vi "CategoricalNB.vi"(8 "error in":errorcluster) -> (0 "error out":errorcluster, 3 "out":refnum<class "CategoricalNB.lvclass">)   [LabVIEW 2020]
doc: "Naive Bayes classifier for categorical features\n\n The categorical Naive Bayes classifier is suitable for classification with\n discrete features that are categorically distributed. The categories of\n each feature are drawn from a categorical distribution.\n\n Read more in the :ref:`User Guide <categorical_naive_bayes>`.\n\n Parameters\n ----------\n alpha : float, default=1.0\n Additive (Laplace/Lidstone) smoothing parameter\n (0 for no smoothing).\n\n fit_prior : bool, default=True\n Whether to learn class prior probabilities or not.\n If false, a uniform prior will be used.\n\n class_prior : array-like of shape (n_classes,), default=None\n Prior probabilities of the classes. If specified the priors are not\n adjusted according to the data.\n\n min_categories : int or array-like of shape (n_features,), default=None\n Minimum number of categories per feature.\n\n - integer: Sets the minimum number of categories per feature to\n `n_categories` for each features.\n - array-like: shape (n_features,) where `n_categories[i]` holds the\n minimum number of categories for the ith column of the input.\n - None (default): Determines the number of categories automatically\n from the training data.\n\n .. versionadded:: 0.24\n\n Attributes\n ----------\n category_count_ : list of arrays of shape (n_features,)\n Holds arrays of shape (n_classes, n_categories of respective feature)\n for each feature. Each array provides the number of samples\n encountered for each class and category of the specific feature.\n\n class_count_ : ndarray of shape (n_classes,)\n Number of samples encountered for each class during fitting. This\n value is weighted by the sample weight when provided.\n\n class_log_prior_ : ndarray of shape (n_classes,)\n Smoothed empirical log probability for each class.\n\n classes_ : ndarray of shape (n_classes,)\n Class labels known to the classifier\n\n feature_log_prob_ : list of arrays of shape (n_features,)\n Holds arrays of shape (n_classes, n_categories of respective feature)\n for each feature. Each array provides the empirical log probability\n of categories given the respective feature and class, ``P(x_i|y)``.\n\n n_features_ : int\n Number of features of each sample.\n\n n_categories_ : ndarray of shape (n_features,), dtype=np.int64\n Number of categories for each feature. This value is\n inferred from the data or set by the minimum number of categories.\n\n .. versionadded:: 0.24\n\n \nAvailable methods:\nFit\nPartial Fit\nPredict\nPredict Log Proba\nPredict Proba\nScore\nGet Attributes\nGet Params\nSet Params"
uses:
  CategoricalNB.lvclass
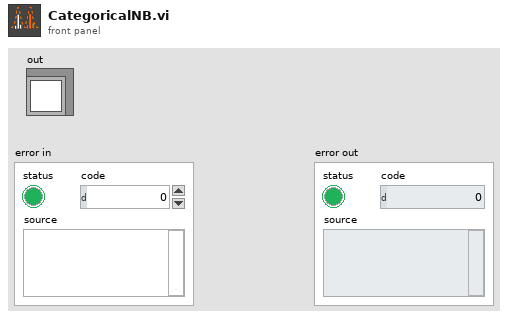
[diagram p1: front panel]
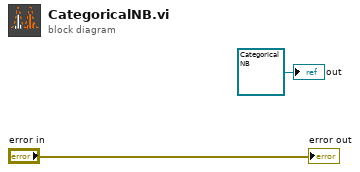
[diagram p0: block diagram]
diagram:
  "out" <- refnum<class "CategoricalNB.lvclass"> refnum ("model")
  "error out" <- "error in"
